vi "Actor Core.vi"(8 "error in":errorcluster, 11 "Receiver in":refnum<class "Receiver.lvclass">) -> (0 "error out":errorcluster, 3 "Actor out":refnum<class "Actor.lvclass">)   [LabVIEW 2013, in "Receiver.lvlib" / "Receiver.lvclass"]
doc: "(<B>Filename</B>: Actor Framework.lvlib:Actor.lvclass:Actor Core.vi)\n\nReceives messages to the actor, reacts to them, and initiates any error handling that may shut the actor down.\n\nDescendant classes may override this VI to append parallel tasks for the actor to complete while it handles messages. Overrides use the Call Parent Method node."
uses:
  Receiver.lvclass
  <vilib>/ActorFramework/Actor/Actor.lvclass
  System/System Status.ctl
  System/SystemStates.ctl
  Command Processor/Command Processor Status.ctl
  Current Previous State Status.ctl
  State Status.ctl
  Command Processor/Command/Command Status.ctl
  Command Processor/Command/State Status.ctl
  Command Processor/Waiting/Waiting.lvclass
  Receiver.lvclass/Receiver.ctl
  <vilib>/ActorFramework/Actor/Actor.lvclass/Actor.ctl
  <vilib>/ActorFramework/Message Enqueuer/Message Enqueuer.lvclass/Message Enqueuer.ctl
  System/System.lvclass
  Receiver Commands Using Processor/Connect Command/Connect Command.lvclass
  Command Processor Messages/Execute Command Msg/Execute Command Msg.lvclass/Execute Command Msg.ctl
  <vilib>/ActorFramework/Message Enqueuer/Init from Existing Queue.vi
  <vilib>/ActorFramework/Message Enqueuer/Enqueue.vi
  <vilib>/ActorFramework/Message Priority Queue/Priority Enqueue.vi
  <vilib>/ActorFramework/Message Enqueuer/Message Enqueuer.lvclass
  Receiver Messages/Go To Not Connected  Msg/Go To Not Connected  Msg.lvclass
  Command Processor Messages/Execute Command Msg/Execute Command Msg.lvclass
  Command Processor Messages/Stop Command Msg/Stop Command Msg.lvclass
  Command Processor/Command Processor.lvclass
  Command Processor/Command/Command.lvclass
panel:
  in  "Execute Connect":bool
  in  "System Status":T1
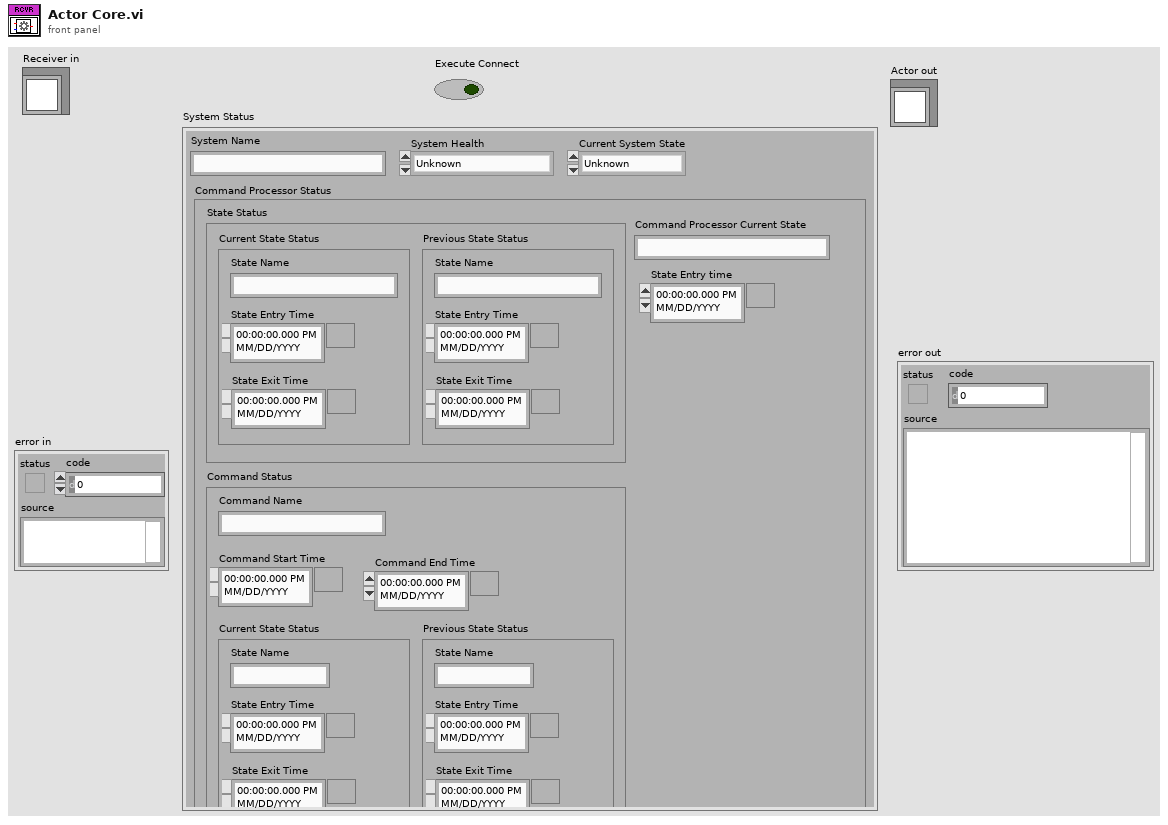
[diagram p1: front panel]
types:
  T1 = typedef "System.lvlib/System.lvclass/System Status.ctl" = cluster{"Current System State":T2, "System Health":enum16{"Unknown", "Good", "Poor", "Bad"}, "System Name":string, "Command Processor Status":T3}
  T2 = typedef "System.lvlib/System.lvclass/SystemStates.ctl" = enum16{"Unknown", "Running", "Stopped"}
  T3 = typedef "Command Processor.lvlib/Command Processor.lvclass/Command Processor Status.ctl" = cluster{"State Entry time":timestamp, "State Status":T4, "Command Processor Current State":string, "Command Status":T6}
  T4 = typedef "Current Previous State Status.ctl" = cluster{"Current State Status":T5, "Previous State Status":T5}
  T5 = typedef "State Status.ctl" = cluster{"State Name":string, "State Entry Time":timestamp, "State Exit Time":timestamp}
  T6 = typedef "Command Processor.lvlib/Command.lvlib/Command.lvclass/Command Status.ctl" = cluster{"Command Name":string, "Current State Status":T7, "Command Start Time":timestamp, "Command End Time":timestamp, "Previous State Status":T7}
  T7 = typedef "Command Processor.lvlib/Command.lvlib/Command.lvclass/State Status.ctl" = cluster{"State Name":string, "State Entry Time":timestamp, "State Exit Time":timestamp}
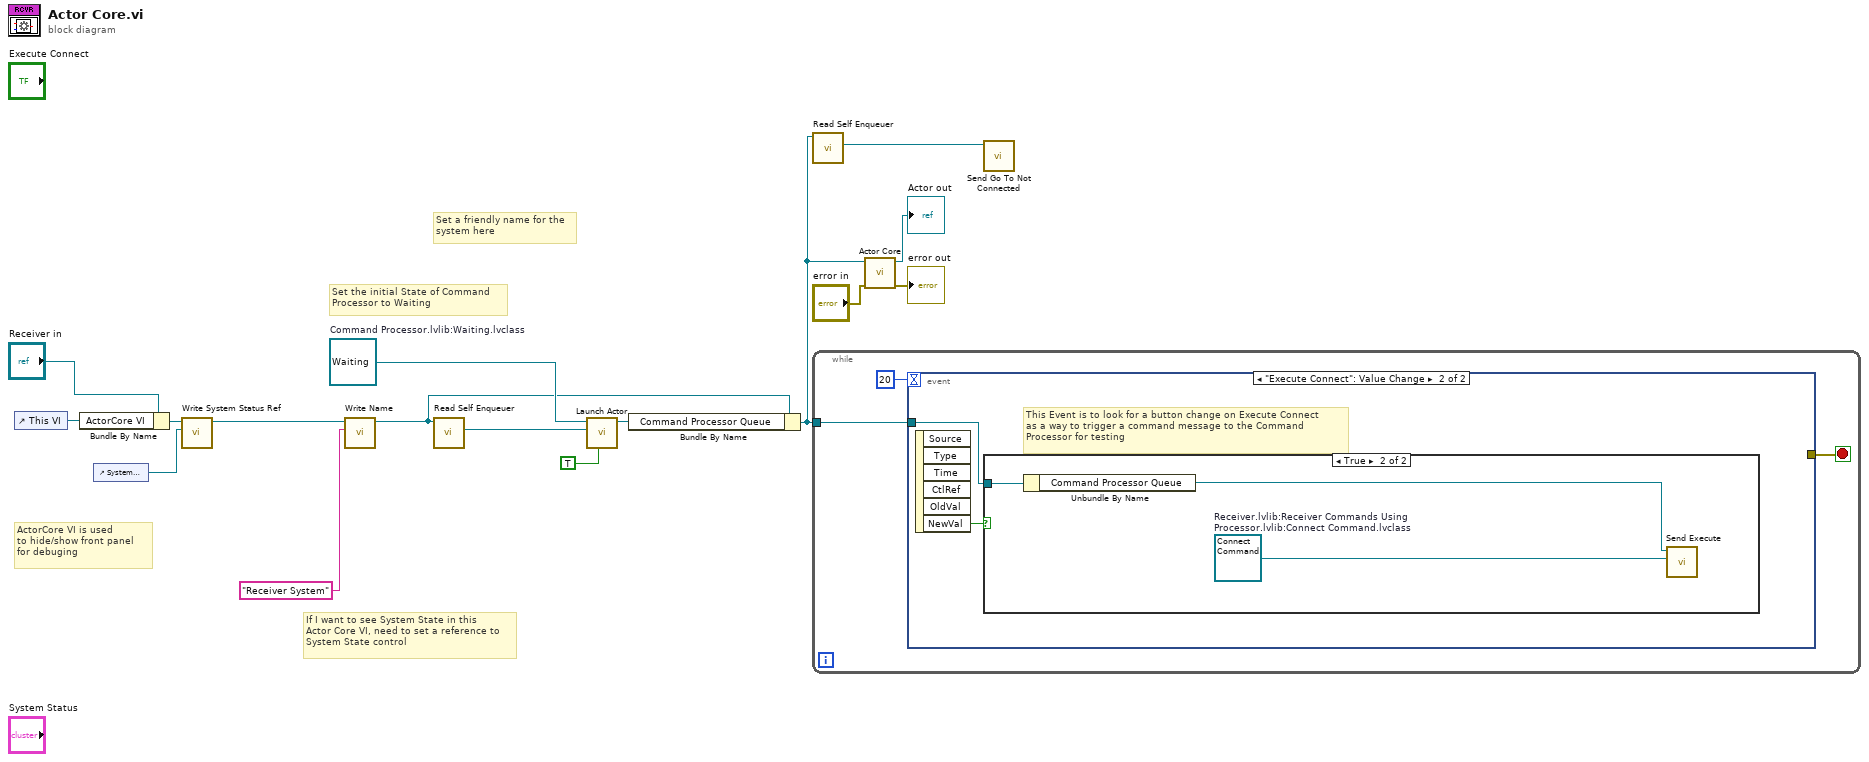
[diagram p0: block diagram]
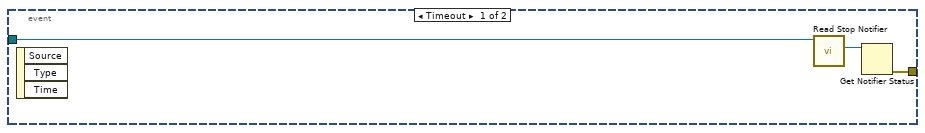
[diagram p2: hidden frame]
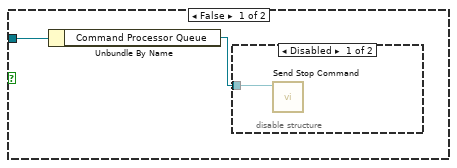
[diagram p3: hidden frame]
diagram:
  w9 = refnum<class "Waiting.lvclass"> refnum  # Command Processor.lvlib:Waiting.lvclass
  # "Set the initial State of Command \nProcessor to Waiting"
  # "Set a friendly name for the\nsystem here"
  # "If I want to see System State in this \nActor Core VI, need to set a reference to\nSystem State control"
  # "ActorCore VI is used\nto hide/show front panel \nfor debuging"
  n1 = control-ref of="This VI"() -> (w14:refnum<vi>)
  n2 = Bundle By Name(cluster="Receiver in", "ActorCore VI"=w14) -> (w6:refnum<class "Receiver.lvclass">)
  n3 = control-ref of="System Status"() -> (w4:refnum<vi>)
  n4 = call-dynamic "Write System Status Ref.vi"("System Status Ref"=w4, "System in"=w6) -> ("System out"=w5:refnum<class "Receiver.lvclass">)  [unwired: 8 in, 1 out]
  n5 = call-dynamic "Write Name.vi"("Name"="Receiver System", "System in"=w5) -> ("System out"=w7:refnum<class "Receiver.lvclass">)  [unwired: 8 in, 1 out]
  n6 = call <vilib>:"Read Self Enqueuer.vi"("Actor"=w7) -> ("Self Enqueuer"=w3:refnum<class "Message Enqueuer.lvclass">)  [unwired: 10 in]
  n7 = call <vilib>:"Launch Actor.vi"("Open Actor Core front panel? (F)"=TRUE, "Actor-to-Caller Enqueuer"=w3, "Actor"=w9) -> ("Caller-To-Actor Enqueuer"=w10:refnum<class "Message Enqueuer.lvclass">)  [unwired: 7 in, 1 out]
  n8 = Bundle By Name(cluster=w7, "Command Processor Queue"=w10) -> (w2:refnum<class "Receiver.lvclass">)
  n9 = call <vilib>:"Read Self Enqueuer.vi"("Actor"=w2) -> ("Self Enqueuer"=w1:refnum<class "Message Enqueuer.lvclass">)  [unwired: 10 in]
  n10 = while {
    tunnel: w2 -> [w18]
    stop <- w17 stop-if-true
    n11 = event shown="[1] \"Execute Connect\": Value Change" {
      selector: _ -> [_ _]
      dyn-events: _ -> [_ _]
      timeout: 20 -> [_ _]
      tunnel: w18 -> [w22 w23]
      tunnel: [w20 _] -> w17
      event Timeout {
        n12 = event-data() -> ()  [unwired: 1 in, 3 out]
        n13 = call-dynamic "Read Stop Notifier.vi"("System in"=w22) -> ("Stop Notifier"=w21:refnum<notifier>)  [unwired: 8 in, 2 out]
        n14 = Get Notifier Status(notifier=w21) -> (error out=w20:errorcluster)  [unwired: 1 in, 4 out]
      }
      event "Execute Connect": Value Change {
        # "This Event is to look for a button change on Execute Connect\nas a way to trigger a command message to the Command\nProcessor for testing"
        n15 = event-data() -> ("NewVal"=w24:bool)  [unwired: 1 in, 5 out]
        n16 = case shown="True" w24 {
          tunnel: w23 -> [w26 w30]
          frame False {
            n17 = Unbundle By Name(w26) -> ("Command Processor Queue"=w25:refnum<class "Message Enqueuer.lvclass">)
            n18 = disable-structure shown="Disabled" {
              disable-tunnel: w25 -> [w27 _]
              frame Disabled {
                n19 = call "Send Stop Command.vi"("Message Enqueuer"=w27) -> ()  [unwired: 9 in, 2 out]
              }
              frame Enabled {
              }
            }
          }
          frame True {
            w28 = refnum<class "Connect Command.lvclass"> refnum  # Receiver.lvlib:Receiver Commands Using Processor.lvlib:Connect Command.lvclass
            n20 = Unbundle By Name(w30) -> ("Command Processor Queue"=w29:refnum<class "Message Enqueuer.lvclass">)
            n21 = call "Send Execute.vi"("Command In"=w28, "Message Enqueuer"=w29) -> ()  [unwired: 8 in, 2 out]
          }
        }
      }
    }
  }
  n22 = call-parent "Actor Core.vi"("error in"="error in", "State in"=w2) -> ("error out"=→"error out":errorcluster, "Actor out"=→"Actor out":refnum<class "Actor.lvclass">)  [unwired: 8 in]
  n23 = call "Send Go To Not Connected .vi"("Message Enqueuer"=w1) -> ()  [unwired: 9 in, 2 out]
